vi "Move_Block_Horizontally.vi"(9 "direction":dbl, 10 "oldBlock":T1 {"orientaion" items=["up", "down", "left", "right"]; "type" items=["t", "rl", "ll", "rz", "lz", "square", "line"]}, 11 "Array":bool[][](array[boolean])) -> (1 "success":bool, 2 "newBlock":T1 {"orientaion" items=["up", "down", "left", "right"]; "type" items=["t", "rl", "ll", "rz", "lz", "square", "line"]})   [LabVIEW 2015]
uses:
  block.ctl
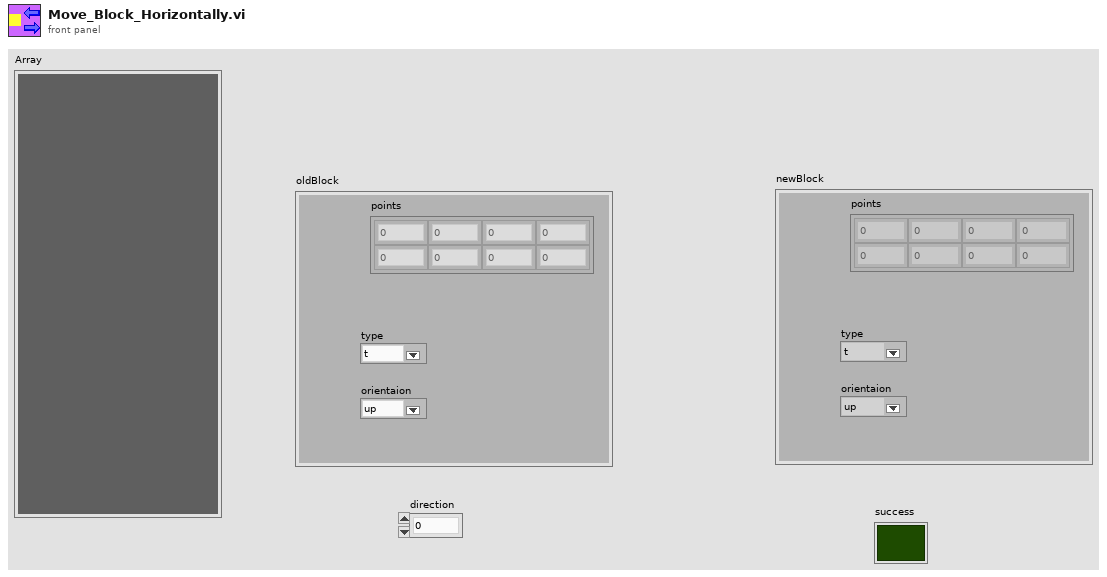
[diagram p1: front panel]
types:
  T1 = typedef "block.ctl" = cluster{"points":dbl[][], "type":u16, "orientaion":u16}
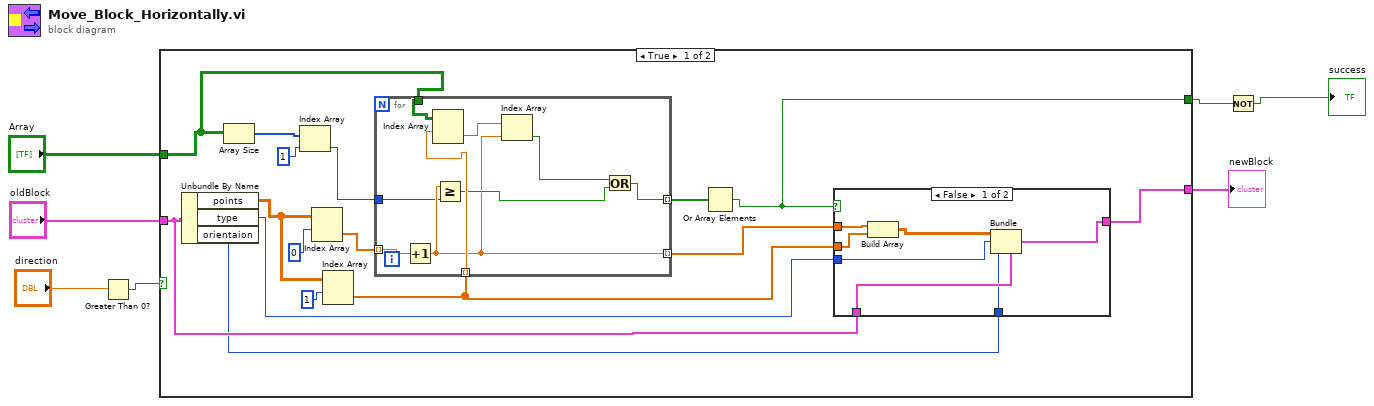
[diagram p0: block diagram]
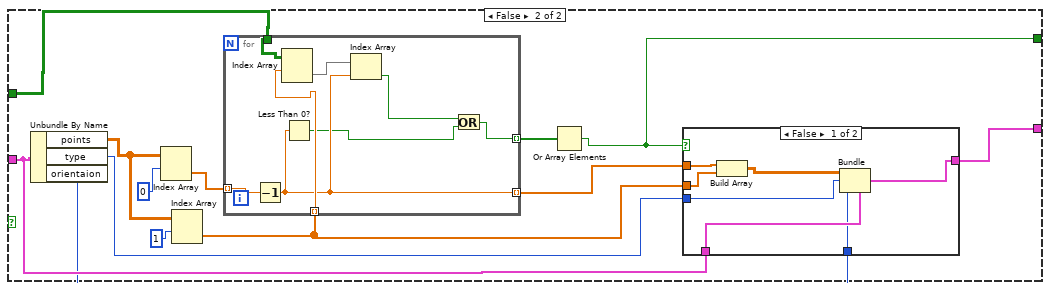
[diagram p3: hidden frame]
diagram:
  n1 = Greater Than 0?(x="direction") -> (x > 0?=w6:bool)
  n2 = case shown="True" w6 {
    tunnel: "oldBlock" -> [w18 w51]
    tunnel: "Array" -> [w12 w45]
    tunnel: [w10 w43] -> w3
    tunnel: [w8 w41] -> w2
    frame True {
      n3 = Unbundle By Name(w18) -> ("points"=w15:dbl[][], "type"=w14:u16, "orientaion"=w13:u16)
      n4 = Array Size(array=w12) -> (size(s)=w20:i32[])
      n5 = Index Array(array=w20, index=1) -> (element=w19:i32)
      n6 = Index Array(array=w15, index (row)=0) -> (element=w22:dbl[])  [unwired: 1 in]
      n7 = Index Array(array=w15, index (row)=1) -> (element=w11:dbl[])  [unwired: 1 in]
      n8 = for {
        tunnel: w22 -> [w32] mode=indexing
        tunnel: [w25] -> w17 mode=indexing
        tunnel: w19 -> [w24]
        tunnel: w11 -> [w30] mode=indexing
        tunnel: w12 -> [w31]
        tunnel: [w26] -> w9 mode=indexing
        n9 = Increment(x=w32) -> (x+1=w25:dbl)
        n10 = Index Array(array=w31, index (row)=w30) -> (element=w29:bool[])  [unwired: 1 in]
        n11 = Greater Or Equal?(x=w25, y=w24) -> (x >= y?=w28:bool)
        n12 = Index Array(array=w29, index=w25) -> (element=w27:bool)
        n13 = Or(x=w27, y=w28) -> (x .or. y?=w26:bool)
      }
      n14 = Or Array Elements(Boolean array=w9) -> (logical OR=w8:bool)
      n15 = case shown="False" w8 {
        tunnel: w18 -> [w36 w40]
        tunnel: [w33 w40] -> w10
        tunnel: w17 -> [w39 _]
        tunnel: w11 -> [w38 _]
        tunnel: w14 -> [w35 _]
        tunnel: w13 -> [w34 _]
        frame False {
          n16 = Build Array(w39, w38) -> (w37:dbl[][])
          n17 = Bundle(cluster=w36, "points"=w37, "type"=w35, "orientaion"=w34) -> (w33:T1)
        }
        frame True {
        }
      }
    }
    frame False {
      n18 = Unbundle By Name(w51) -> ("points"=w48:dbl[][], "type"=w47:u16, "orientaion"=w46:u16)
      n19 = Index Array(array=w48, index (row)=0) -> (element=w52:dbl[])  [unwired: 1 in]
      n20 = Index Array(array=w48, index (row)=1) -> (element=w44:dbl[])  [unwired: 1 in]
      n21 = for {
        tunnel: w52 -> [w61] mode=indexing
        tunnel: [w57] -> w50 mode=indexing
        tunnel: w44 -> [w59] mode=indexing
        tunnel: w45 -> [w60]
        tunnel: [w54] -> w42 mode=indexing
        n22 = Decrement(x=w61) -> (x-1=w57:dbl)
        n23 = Index Array(array=w60, index (row)=w59) -> (element=w58:bool[])  [unwired: 1 in]
        n24 = Less Than 0?(x=w57) -> (x < 0?=w56:bool)
        n25 = Index Array(array=w58, index=w57) -> (element=w55:bool)
        n26 = Or(x=w55, y=w56) -> (x .or. y?=w54:bool)
      }
      n27 = Or Array Elements(Boolean array=w42) -> (logical OR=w41:bool)
      n28 = case shown="False" w41 {
        tunnel: w51 -> [w65 w69]
        tunnel: [w62 w69] -> w43
        tunnel: w50 -> [w68 _]
        tunnel: w44 -> [w67 _]
        tunnel: w47 -> [w64 _]
        tunnel: w46 -> [w63 _]
        frame False {
          n29 = Build Array(w68, w67) -> (w66:dbl[][])
          n30 = Bundle(cluster=w65, "points"=w66, "type"=w64, "orientaion"=w63) -> (w62:T1)
        }
        frame True {
        }
      }
    }
  }
  "newBlock" <- w3
  n31 = Not(x=w2) -> (.not. x?=→"success":bool)
